vi "Set caption.vi"(9 "index (row)":i32, 10 "Array":string[][](array[string]), 11 "Control in":refnum<vi>) -> (0 "error out":errorcluster, 3 "reference out":refnum<vi>)   [LabVIEW 2019]
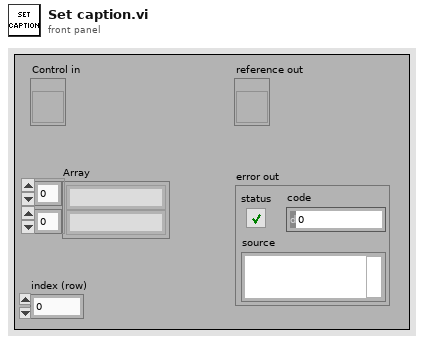
[diagram p1: front panel]
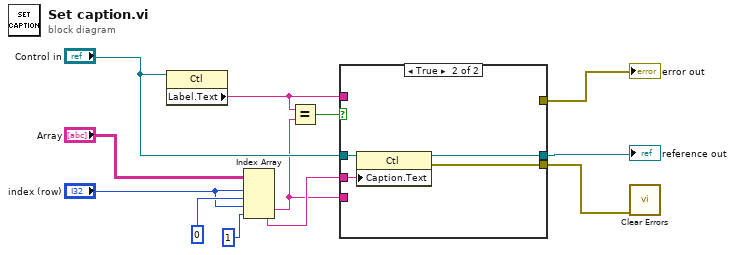
[diagram p0: block diagram]
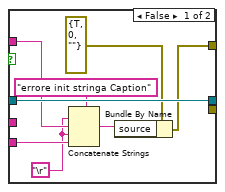
[diagram p2: hidden frame]
diagram:
  n1 = property on="Property Node" class="Ctl"(reference="Control in") -> ("Label.Text"=w2:string)  [unwired: 1 in, 2 out]
  n2 = Index Array(array="Array", index (row) #1="index (row)", index (col) #1=0 ("index (row)"), index (row) #2="index (row)", index (col) #2=1 ("disabled index (col)")) -> (element #1=w1:string, element #2=w11:string)
  n3 = Equal?(x=w2, y=w1) -> (x = y?=w4:bool)
  n4 = case shown="True" w4 {
    tunnel: [_ w24] -> w12
    tunnel: w11 -> [_ w23]
    tunnel: [w20 w22] -> w8
    tunnel: "Control in" -> [w20 w21]
    tunnel: [w18 _] -> w3
    tunnel: w2 -> [w16 _]
    tunnel: w1 -> [w15 _]
    frame False {
      w14 = "\r"
      n5 = Concatenate Strings("errore init stringa Caption" ("string"), w14, w16, w14, w15) -> (w17:string)
      n6 = Bundle By Name(cluster=errorcluster {"status"=TRUE, "code"=0, "source"=""} ("error out"), "source"=w17) -> (w18:errorcluster)
    }
    frame True {
      n7 = property class="Ctl"(reference=w21, "Caption.Text"=w23) -> (reference out=w22:refnum<vi>, error out=w24:errorcluster)  [unwired: 1 in]
    }
  }
  "reference out" <- w8
  "error out" <- w3
  n8 = call <vilib>:"Clear Errors.vi"("error in (no error)"=w12) -> ()  [unwired: 5 in, 2 out]
